vi "15TMonitor.vi"() -> ()   [LabVIEW 2019]
uses:
  Utility/Monitor Communication/Berta/15T-Cluster.ctl
  Global/Global Variables/Data_Display_global.vi
  Instrument_Setup.vi
panel:
  out "15T-Cluster":T1={"Magnet (T)"=0.0, "Leads (T)"=0.0, "Setpoint (T)"=3.4572, "Rate (T/min)"=0.0, "Set"=FALSE, "Zero"=FALSE, "Hold"=FALSE, "Go to zero"=FALSE, "Go to Hold"=FALSE, "Go to Set"=FALSE, "Clamp"=FALSE, "Switch Heater"=FALSE, "Rate limit"=FALSE, "Switch"=FALSE, "Clamped"=FALSE, "Persistent"=FALSE, "Quenched"=FALSE, "Sweeping"=FALSE, "Select"=FALSE} {"Rate (T/min)" format="%6_5f"; "Setpoint (T)" format="%6_5f"}
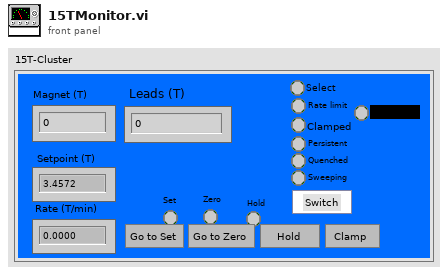
[diagram p1: front panel]
types:
  T1 = typedef "15T-Cluster.ctl" = cluster{"Magnet (T)":dbl, "Leads (T)":dbl, "Setpoint (T)":dbl, "Rate (T/min)":dbl, "Set":bool, "Zero":bool, "Hold":bool, "Go to zero":bool, "Go to Hold":bool, "Go to Set":bool, "Clamp":bool, "Switch Heater":bool, "Rate limit":bool, "Switch":bool, "Clamped":bool, "Persistent":bool, "Quenched":bool, "Sweeping":bool, "Select":bool}
  T2 = typedef "PSIO.ctl" = cluster{"Address":T3, "Version":enum16{"PS", "IPS"}}
  T3 = typedef "OxfordAddress.ctl" = cluster{"Com Port":i32, "ISOBUS Address":i32, "GPIB Address":i16, "Communication":enum16{"RS232", "ISOBUS", "GPIB", "Gateway"}}
  T4 = cluster{"Version\n":string, "Max Sweep":dbl[unit], "Max Field":dbl[unit], "IO Info":T2, "Switch htr dly":dbl[unit]}
  T5 = cluster{"Value":i16, "At rest":bool, "Sweeping":bool, "Rate limiting":bool}
  T6 = cluster{"Value":i16, "Hold":bool, "To set point":bool, "To zero":bool, "Clamped":bool}
  T7 = cluster{"Value":i16, "Off (at zero field)":bool, "On":bool, "Off (at field)":bool, "No switch fitted":bool, "Confirm":bool}
  T8 = cluster{"Value":i16, "Desired":u16, "Magnet":u16, "Commanded":u16, "Actual":u16}
  T9 = cluster{"Value":i16, "Quenched":bool, "Over heated":bool, "Warming up":bool}
  T10 = typedef "15T-Control.ctl" = cluster{"Setpoint (T)":dbl, "Rate (T/min)":dbl, "Go to zero":bool, "Go to Hold":bool, "Go to Set":bool, "Clamp":bool, "Switch Heater":bool}
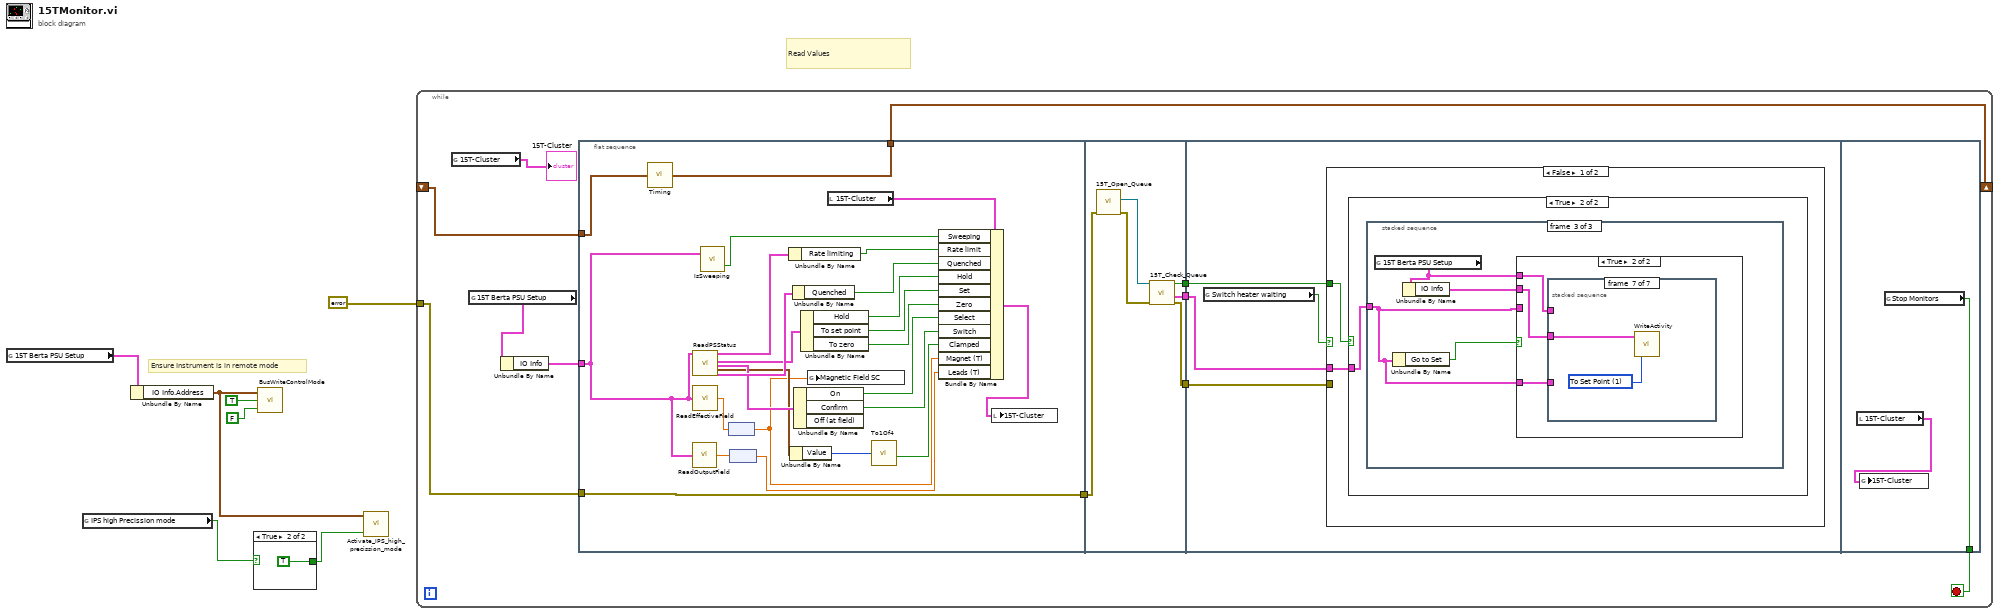
[diagram p0: block diagram]
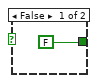
[diagram p2: hidden frame]
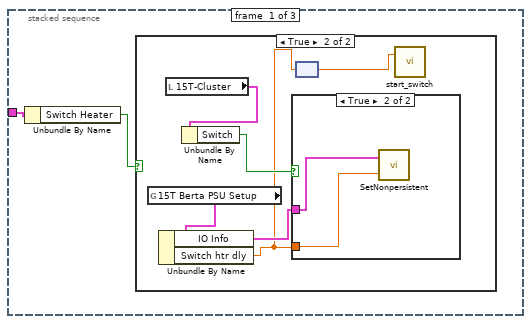
[diagram p4: hidden frame]
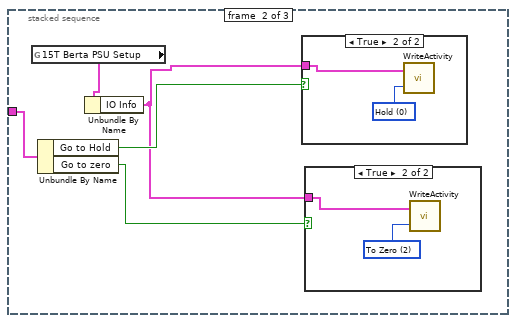
[diagram p7: hidden frame]
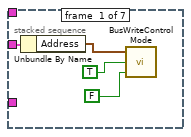
[diagram p11: hidden frame]
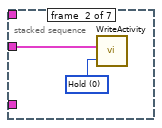
[diagram p12: hidden frame]
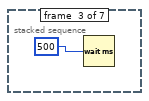
[diagram p13: hidden frame]
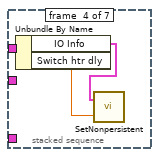
[diagram p14: hidden frame]
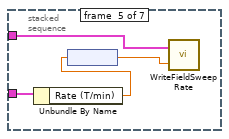
[diagram p15: hidden frame]
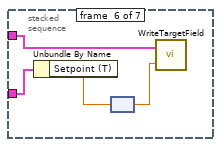
[diagram p16: hidden frame]
diagram:
  # "Read Values"
  # "Ensure Instrument is in remote mode"
  n1 = global read "Instrument_Setup.vi" "15T Berta PSU Setup"() -> (w6:T4)
  n2 = global read "Instrument_Setup.vi" "IPS high Precission mode"() -> (w2:bool)
  n3 = Unbundle By Name(w6) -> ("IO Info.Address"=w1:T3)
  n4 = case shown="True" w2 {
    tunnel: [FALSE TRUE] -> w3
    frame False {
    }
    frame True {
    }
  }
  n5 = call "BusWriteControlMode.vi"("Locked"=FALSE, "Remote"=TRUE, "Address"=w1) -> ()  [unwired: 1 out]
  n6 = call "Activate_IPS_high_precission_mode.vi"("High Precission"=w3, "Address"=w1) -> ()  [unwired: 1 in, 1 out]
  n7 = while {
    tunnel: errorcluster {"status"=FALSE, "code"=0, "source"=""} ("error in (no error)") -> [w19]
    shift-right: [w17] -> _
    shift-left: _ -> [w18]
    stop <- w14 stop-if-true
    n8 = global read "Data_Display_global.vi" "15T-Cluster"() -> (→"15T-Cluster":T1)
    n9 = global read "Instrument_Setup.vi" "15T Berta PSU Setup"() -> (w16:T4)
    n10 = Unbundle By Name(w16) -> ("IO Info"=w15:T2)
    n11 = flat-sequence {
      tunnel: w19 -> [w21]
      tunnel: w18 -> [w45]
      tunnel: [w44] -> w17
      tunnel: w15 -> [w43]
      tunnel: [w21] -> w13
      tunnel: w13 -> [w51]
      tunnel: [w48] -> w12
      tunnel: [w47] -> w11
      tunnel: [w46] -> w10
      tunnel: w12 -> [w54]
      tunnel: w11 -> [w53]
      tunnel: w10 -> [w52]
      tunnel: [w106] -> w14
      frame #0 {
        n12 = call "Timing.vi"("start time (s)"=w45) -> ("last reading (s)"=w44:timestamp)
        n13 = call "ReadOutputField.vi"("IO Info"=w43) -> ("Field"=w41:dbl[unit])  [unwired: 2 out]
        n14 = call "ReadPSStatus.vi"("IO Info"=w43) -> ("Mode (n)"=w40:T5, "Activity"=w38:T6, "Switch Heater"=w37:T7, "Polarity"=w36:T8, "System Status (m)"=w39:T9)  [unwired: 10 in, 4 out]
        n15 = call "ReadEffectiveField.vi"("IO Info"=w43) -> ("Effective field"=w42:dbl[unit])  [unwired: 2 out]
        n16 = call "IsSweeping.vi"("IO Info"=w43) -> ("Sweeping"=w32:bool)  [unwired: 1 in, 1 out]
        n17 = node(w42) -> (w22:dbl)
        n18 = node(w41) -> (w23:dbl)
        n19 = Unbundle By Name(w40) -> ("Rate limiting"=w31:bool)
        n20 = Unbundle By Name(w36) -> ("Value"=w35:i16)
        n21 = Unbundle By Name(w39) -> ("Quenched"=w30:bool)
        n22 = Unbundle By Name(w37) -> ("On"=w26:bool, "Confirm"=w25:bool)  [unwired: 1 out]
        n23 = Unbundle By Name(w38) -> ("Hold"=w29:bool, "To set point"=w28:bool, "To zero"=w27:bool)
        n24 = global write "Data_Display_global.vi" "Magnetic Field SC"(w22) -> ()
        n25 = local read "15T-Cluster"() -> (w34:T1)
        n26 = call "To1Of4.vi"("Input"=w35) -> ("3"=w24:bool)  [unwired: 3 out]
        n27 = Bundle By Name(cluster=w34, "Sweeping"=w32, "Rate limit"=w31, "Quenched"=w30, "Hold"=w29, "Set"=w28, "Zero"=w27, "Select"=w26, "Switch"=w25, "Clamped"=w24, "Magnet (T)"=w22, "Leads (T)"=w23) -> (w33:T1)
        n28 = local write "15T-Cluster"(w33) -> ()
      }
      frame #1 {
        n29 = call "15T_Open_Queue.vi"("error in (no error)"=w51) -> ("error out"=w49:errorcluster, "queue out"=w50:refnum<queue>)  [unwired: 9 in]
        n30 = call "15T_Check_Queue.vi"("error in (no error)"=w49, "queue"=w50) -> ("error out"=w48:errorcluster, "15T-Control"=w46:T10, "New Entries?"=w47:bool)  [unwired: 6 in]
      }
      frame #2 {
        n31 = global read "Data_Display_global.vi" "Switch heater waiting"() -> (w55:bool)
        n32 = case shown="False" w55 {
          tunnel: w54 -> [_ _]
          tunnel: w53 -> [w57 _]
          tunnel: w52 -> [w56 _]
          frame False {
            n33 = case shown="True" w57 {
              tunnel: w56 -> [_ w58]
              frame False {
              }
              frame True {
                n34 = stacked-sequence {
                  tunnel: w58 -> [w60 w73 w78]
                  frame #0 {
                    n35 = Unbundle By Name(w60) -> ("Switch Heater"=w59:bool)
                    n36 = case shown="True" w59 {
                      frame False {
                      }
                      frame True {
                        n37 = global read "Instrument_Setup.vi" "15T Berta PSU Setup"() -> (w64:T4)
                        n38 = Unbundle By Name(w64) -> ("IO Info"=w63:T2, "Switch htr dly"=w62:dbl[unit])
                        n39 = local read "15T-Cluster"() -> (w66:T1)
                        n40 = Unbundle By Name(w66) -> ("Switch"=w65:bool)
                        n41 = case shown="True" w65 {
                          tunnel: w62 -> [_ w68]
                          tunnel: w63 -> [_ w67]
                          frame False {
                          }
                          frame True {
                            n42 = call "SetNonpersistent.vi"("Switch Heater Dwell Time"=w68, "IO Info"=w67) -> ()  [unwired: 2 out]
                          }
                        }
                        n43 = node(w62) -> (w61:dbl)
                        n44 = call "start_switch.vi"("Switch heater time"=w61) -> ()  [unwired: 2 in]
                      }
                    }
                  }
                  frame #1 {
                    n45 = global read "Instrument_Setup.vi" "15T Berta PSU Setup"() -> (w72:T4)
                    n46 = Unbundle By Name(w73) -> ("Go to Hold"=w71:bool, "Go to zero"=w70:bool)
                    n47 = Unbundle By Name(w72) -> ("IO Info"=w69:T2)
                    n48 = case shown="True" w71 {
                      tunnel: w69 -> [_ w76]
                      frame False {
                      }
                      frame True {
                        w77 = u16 0 items=["Hold", "To Set Point", "To Zero", "Clamp"] ("Activity")
                        n49 = call "WriteActivity.vi"("Activity"=w77, "IO Info"=w76) -> ()  [unwired: 1 in, 1 out]
                      }
                    }
                    n50 = case shown="True" w70 {
                      tunnel: w69 -> [_ w74]
                      frame False {
                      }
                      frame True {
                        w75 = u16 2 items=["Hold", "To Set Point", "To Zero", "Clamp"] ("Activity")
                        n51 = call "WriteActivity.vi"("Activity"=w75, "IO Info"=w74) -> ()  [unwired: 1 in, 1 out]
                      }
                    }
                  }
                  frame #2 {
                    n52 = global read "Instrument_Setup.vi" "15T Berta PSU Setup"() -> (w79:T4)
                    n53 = Unbundle By Name(w78) -> ("Go to Set"=w81:bool)
                    n54 = Unbundle By Name(w79) -> ("IO Info"=w80:T2)
                    n55 = case shown="True" w81 {
                      tunnel: w78 -> [_ _]
                      tunnel: w80 -> [_ w84]
                      tunnel: w79 -> [_ w83]
                      tunnel: w78 -> [_ w82]
                      frame False {
                      }
                      frame True {
                        n56 = stacked-sequence {
                          tunnel: w84 -> [w88 w89 _ _ w95 w99 w103]
                          tunnel: w83 -> [_ _ _ w94 _ _ _]
                          tunnel: w82 -> [_ _ _ _ w98 w102 _]
                          frame #0 {
                            n57 = Unbundle By Name(w88) -> ("Address"=w87:T3)
                            n58 = call "BusWriteControlMode.vi"("Locked"=FALSE, "Remote"=TRUE, "Address"=w87) -> ()  [unwired: 1 out]
                          }
                          frame #1 {
                            w90 = u16 0 items=["Hold", "To Set Point", "To Zero", "Clamp"] ("Activity")
                            n59 = call "WriteActivity.vi"("Activity"=w90, "IO Info"=w89) -> ()  [unwired: 1 in, 1 out]
                          }
                          frame #2 {
                            n60 = Wait (ms)(milliseconds to wait=500) -> ()  [unwired: 1 out]
                          }
                          frame #3 {
                            n61 = Unbundle By Name(w94) -> ("IO Info"=w92:T2, "Switch htr dly"=w93:dbl[unit])
                            n62 = call "SetNonpersistent.vi"("Switch Heater Dwell Time"=w93, "IO Info"=w92) -> ()  [unwired: 2 out]
                          }
                          frame #4 {
                            n63 = Unbundle By Name(w98) -> ("Rate (T/min)"=w97:dbl)
                            n64 = node(w97) -> (w96:dbl[unit])
                            n65 = call "WriteFieldSweepRate.vi"("Sweep rate"=w96, "IO Info"=w95) -> ()  [unwired: 1 out]
                          }
                          frame #5 {
                            n66 = Unbundle By Name(w102) -> ("Setpoint (T)"=w101:dbl)
                            n67 = node(w101) -> (w100:dbl[unit])
                            n68 = call "WriteTargetField.vi"("Target Field"=w100, "IO Info"=w99) -> ()  [unwired: 1 in, 1 out]
                          }
                          frame #6 {
                            w104 = u16 1 items=["Hold", "To Set Point", "To Zero", "Clamp"] ("Activity")
                            n69 = call "WriteActivity.vi"("Activity"=w104, "IO Info"=w103) -> ()  [unwired: 1 in, 1 out]
                          }
                        }
                      }
                    }
                  }
                }
              }
            }
          }
          frame True {
          }
        }
      }
      frame #3 {
        n70 = local read "15T-Cluster"() -> (w105:T1)
        n71 = global write "Data_Display_global.vi" "15T-Cluster"(w105) -> ()
        n72 = global read "Data_Display_global.vi" "Stop Monitors"() -> (w106:bool)
      }
    }
  }
